vi "CmdexLedCps.vi"(0 "Error Input":errorcluster, 5 "LED Id":enum16{"LED0", "LED1", "LED2", "LED3"}(ring), 7 "Width (ms)":u16, 9 "Period (ms)":u16=50, 11 "Uart Input":cluster{u64}={1768843040} {"?" format="%x"}, 12 "Delay (ms)":u16) -> (4 "Error Output":errorcluster, 15 "Uart Output":cluster{u64}={1768843040} {"?" format="%x"})   [LabVIEW 2019]
doc: "<B>Cmdex</B>\nGenerate clock-pulse on the LED."
uses:
  dll/LabViewUart.dll
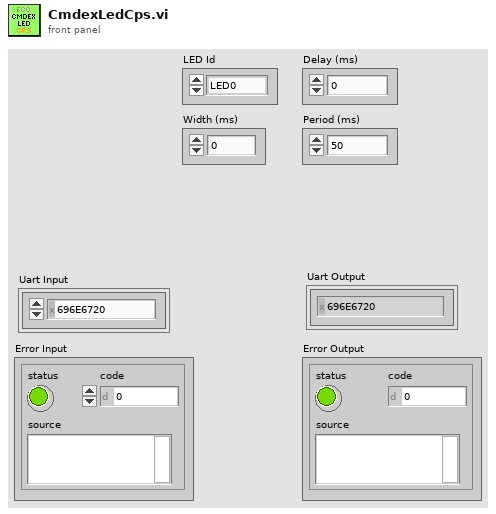
[diagram p1: front panel]
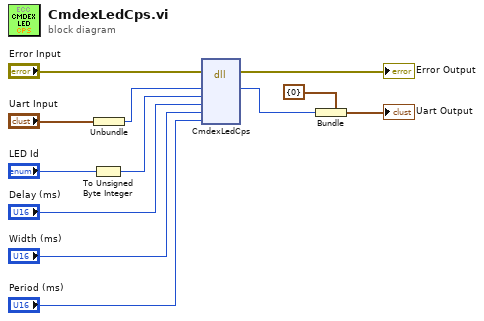
[diagram p0: block diagram]
diagram:
  n1 = To Unsigned Byte Integer(number="LED Id") -> (unsigned 8bit integer=w7:u8)
  n2 = Unbundle("Uart Input") -> (w9:u64)
  n3 = dll-call lib="D:/Google Drive/INC-2020/INC352/INC352-2020/LabVIEW/examples/uart-cmdex/SubVI/dll/LabViewUart.dll" fn="CmdexLedCps"(error in="Error Input", "Uart Handle"=w9, "id"=w7, "delay"="Delay (ms)", "width"="Width (ms)", "period"="Period (ms)") -> (error out=→"Error Output":errorcluster, "Uart Handle"=w3:u64)  [unwired: 7 in, 1 out]
  n4 = Bundle(cluster=cluster{u64} {0}, w3) -> (→"Uart Output":cluster{u64})
